vi "FlatToRichnixnet_grpc_SetSubPropertyRequest.vi"(5 "OutputClusterType":T1, 11 "InputCluster":T3) -> (3 "OutputCluster":T1)   [LabVIEW 2025, in "grpc-xnet_client.lvlib"]
uses:
  nixnet_grpc_SetSubPropertyRequest_Flat.ctl
  nidevice_grpc_Session_Flat.ctl
  nixnet_grpc_SubProperty.ctl
  nixnet_grpc_SetSubPropertyRequest.ctl
  nixnet_grpc_SetSubPropertyRequest_subproperty_id_enum/nixnet_grpc_SetSubPropertyRequest_subproperty_id_enum.lvclass
  nixnet_grpc_SetSubPropertyRequest_property_value/nixnet_grpc_SetSubPropertyRequest_property_value.lvclass
  nidevice_grpc_Session.ctl
  grpc-xnet_client.lvlib
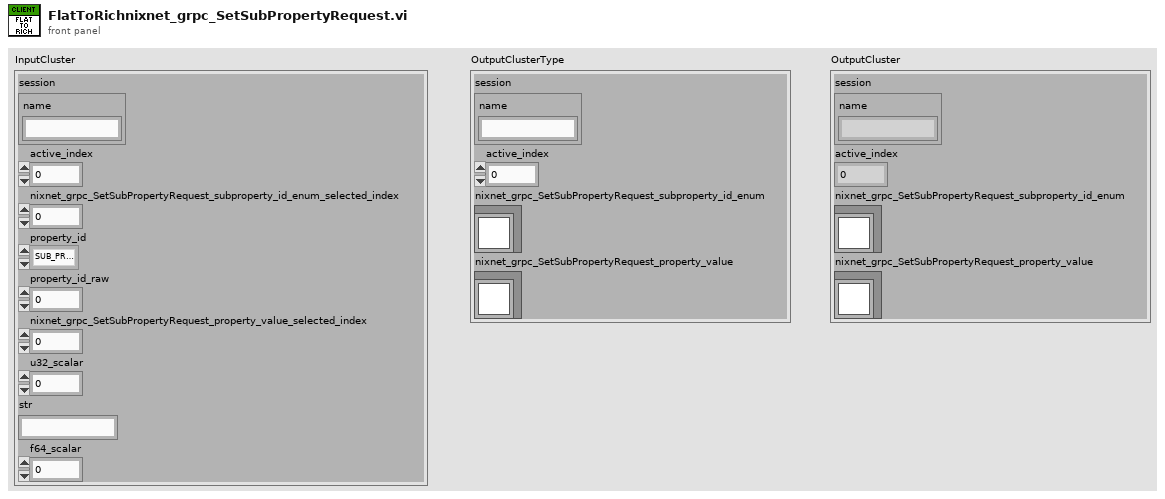
[diagram p1: front panel]
types:
  T1 = typedef "grpc-xnet_client.lvlib/nixnet_grpc_SetSubPropertyRequest.ctl" = cluster{"session":T2, "active_index":u32, "nixnet_grpc_SetSubPropertyRequest_subproperty_id_enum":refnum<class "nixnet_grpc_SetSubPropertyRequest_subproperty_id_enum.lvclass">, "nixnet_grpc_SetSubPropertyRequest_property_value":refnum<class "nixnet_grpc_SetSubPropertyRequest_property_value.lvclass">}
  T2 = typedef "grpc-xnet_client.lvlib/nidevice_grpc_Session.ctl" = cluster{"name":string}
  T3 = typedef "grpc-xnet_client.lvlib/nixnet_grpc_SetSubPropertyRequest_Flat.ctl" = cluster{"session":T4, "active_index":u32, "nixnet_grpc_SetSubPropertyRequest_subproperty_id_enum_selected_index":i32, "property_id":T5, "property_id_raw":u32, "nixnet_grpc_SetSubPropertyRequest_property_value_selected_index":i32, "u32_scalar":u32, "str":string, "f64_scalar":dbl}
  T4 = typedef "grpc-xnet_client.lvlib/nidevice_grpc_Session_Flat.ctl" = cluster{"name":string}
  T5 = typedef "grpc-xnet_client.lvlib/nixnet_grpc_SubProperty.ctl" = enum32{"SUB_PROPERTY_UNSPECIFIED", "SUB_PROPERTY_SESSION_SUB_CAN_START_TIME_OFF", "SUB_PROPERTY_SESSION_SUB_CAN_TX_TIME", "SUB_PROPERTY_SESSION_SUB_LIN_TX_N_CORRUPTED_CHKSUMS", "SUB_PROPERTY_SESSION_SUB_OUTPUT_QUEUE_UPDATE_FREQ", "SUB_PROPERTY_SESSION_SUB_J1939_ADDR_FILTER", "SUB_PROPERTY_SESSION_SUB_SKIP_N_CYCLIC_FRAMES"}
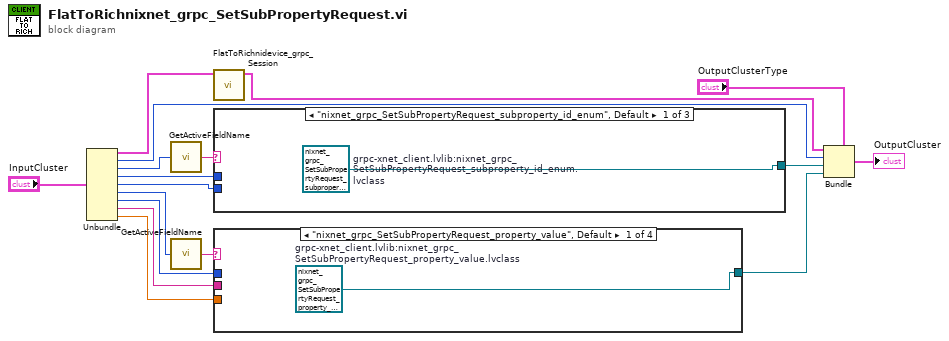
[diagram p0: block diagram]
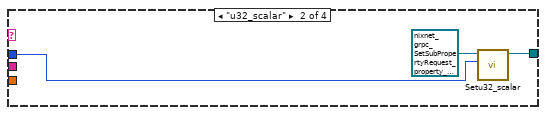
[diagram p2: hidden frame]
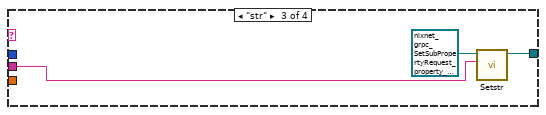
[diagram p3: hidden frame]
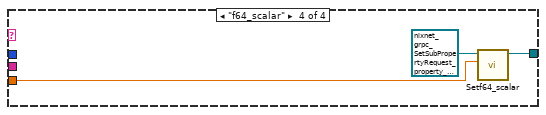
[diagram p4: hidden frame]
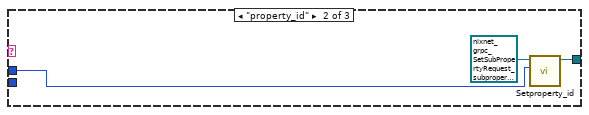
[diagram p5: hidden frame]
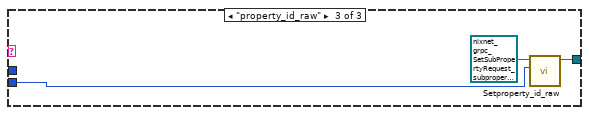
[diagram p6: hidden frame]
diagram:
  n1 = Unbundle "Unbundle"("InputCluster") -> ("session"=w14:T4, "active_index"=w12:u32, "nixnet_grpc_SetSubPropertyRequest_subproperty_id_enum_selected_index"=w11:i32, "property_id"=w8:T5, "property_id_raw"=w7:u32, "nixnet_grpc_SetSubPropertyRequest_property_value_selected_index"=w6:i32, "u32_scalar"=w3:u32, "str"=w2:string, "f64_scalar"=w1:dbl)
  n2 = call "GetActiveFieldName.vi"("protobuf index"=w11) -> ("oneof field name"=w10:string)
  n3 = call "GetActiveFieldName.vi"("protobuf index"=w6) -> ("oneof field name"=w5:string)
  n4 = call "FlatToRichnidevice_grpc_Session.vi"("InputCluster"=w14) -> ("OutputCluster"=w13:T2)  [unwired: 10 in]
  n5 = case "nixnet_grpc_SetSubPropertyRequest_subproperty_id_enum" shown="\"nixnet_grpc_SetSubPropertyRequest_subproperty_id_enum\", Default" w10 {
    tunnel: [w18 w20 w23] -> w9
    tunnel: w8 -> [_ w21 _]
    tunnel: w7 -> [_ _ w24]
    frame "nixnet_grpc_SetSubPropertyRequest_subproperty_id_enum", Default {
      w18 = refnum<class "nixnet_grpc_SetSubPropertyRequest_subproperty_id_enum.lvclass"> refnum  # grpc-xnet_client.lvlib:nixnet_grpc_SetSubPropertyRequest_subproperty_id_enum.lvclass
    }
    frame "property_id" {
      n6 = call "Setproperty_id.vi"("Set_Val"=w21, "OneOfTemplate in"=refnum<class "nixnet_grpc_SetSubPropertyRequest_subproperty_id_enum.lvclass"> refnum) -> ("OneOfTemplate out"=w20:refnum<class "nixnet_grpc_SetSubPropertyRequest_subproperty_id_enum.lvclass">)  [unwired: 8 in, 1 out]
    }
    frame "property_id_raw" {
      n7 = call "Setproperty_id_raw.vi"("Set_Val"=w24, "OneOfTemplate in"=refnum<class "nixnet_grpc_SetSubPropertyRequest_subproperty_id_enum.lvclass"> refnum) -> ("OneOfTemplate out"=w23:refnum<class "nixnet_grpc_SetSubPropertyRequest_subproperty_id_enum.lvclass">)  [unwired: 8 in, 1 out]
    }
  }
  n8 = case "nixnet_grpc_SetSubPropertyRequest_property_value" shown="\"nixnet_grpc_SetSubPropertyRequest_property_value\", Default" w5 {
    tunnel: [w25 w27 w30 w33] -> w4
    tunnel: w3 -> [_ w28 _ _]
    tunnel: w2 -> [_ _ w31 _]
    tunnel: w1 -> [_ _ _ w34]
    frame "nixnet_grpc_SetSubPropertyRequest_property_value", Default {
      w25 = refnum<class "nixnet_grpc_SetSubPropertyRequest_property_value.lvclass"> refnum  # grpc-xnet_client.lvlib:nixnet_grpc_SetSubPropertyRequest_property_value.lvclass
    }
    frame "u32_scalar" {
      n9 = call "Setu32_scalar.vi"("Set_Val"=w28, "OneOfTemplate in"=refnum<class "nixnet_grpc_SetSubPropertyRequest_property_value.lvclass"> refnum) -> ("OneOfTemplate out"=w27:refnum<class "nixnet_grpc_SetSubPropertyRequest_property_value.lvclass">)  [unwired: 8 in, 1 out]
    }
    frame "str" {
      n10 = call "Setstr.vi"("Set_Val"=w31, "OneOfTemplate in"=refnum<class "nixnet_grpc_SetSubPropertyRequest_property_value.lvclass"> refnum) -> ("OneOfTemplate out"=w30:refnum<class "nixnet_grpc_SetSubPropertyRequest_property_value.lvclass">)  [unwired: 8 in, 1 out]
    }
    frame "f64_scalar" {
      n11 = call "Setf64_scalar.vi"("Set_Val"=w34, "OneOfTemplate in"=refnum<class "nixnet_grpc_SetSubPropertyRequest_property_value.lvclass"> refnum) -> ("OneOfTemplate out"=w33:refnum<class "nixnet_grpc_SetSubPropertyRequest_property_value.lvclass">)  [unwired: 8 in, 1 out]
    }
  }
  n12 = Bundle "Bundle"(cluster="OutputClusterType", "session"=w13, "active_index"=w12, "nixnet_grpc_SetSubPropertyRequest_subproperty_id_enum"=w9, "nixnet_grpc_SetSubPropertyRequest_property_value"=w4) -> (→"OutputCluster":T1)
